vi "Enqueue FGV.vi"(8 "error in (no error)":errorcluster, 9 "Dato":variant, 10 "Mensaje":string, 11 "Modulo a obtener":T1) -> (0 "error out":errorcluster)   [LabVIEW 2018, in "Mensajes.lvlib"]
uses:
  Mensajes.lvlib
  Controles/Lista Modulos.ctl
  Controles/FGV Opciones.ctl
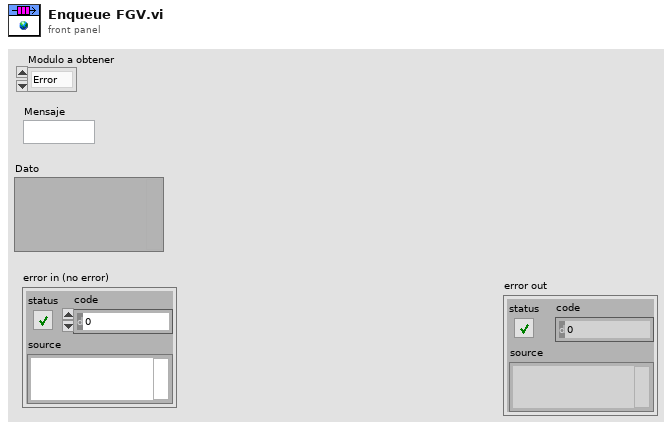
[diagram p1: front panel]
types:
  T1 = typedef "Lista Modulos.ctl" = enum16{"Error", "UI", "Controler", "Config", "Database"}
  T2 = typedef "FGV Opciones.ctl" = enum16{"Get", "Create", "Destroy"}
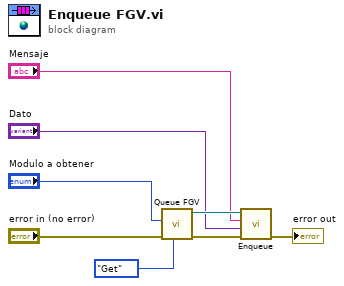
[diagram p0: block diagram]
diagram:
  n1 = call "Queue FGV.vi"("Enum"=FGV_Opciones."Get", "error in (no error)"="error in (no error)", "Modulo a obtener"="Modulo a obtener") -> ("error out"=w5:errorcluster, "Queue Ref"=w6:refnum<queue>)  [unwired: 7 in]
  n2 = call "Enqueue.vi"("error in (no error)"=w5, "Dato"="Dato", "Mensaje"="Mensaje", "Queue in"=w6) -> ("error out"=→"error out":errorcluster)  [unwired: 7 in]
